vi "Dashboard Main.vi"() -> ()   [LabVIEW 2012]
uses:
  <vilib>/event_ctls.llb/eventvkey.ctl
  <vilib>/Utility/config.llb/Read Key (String).vi
  <vilib>/Utility/config.llb/Read Key (I32).vi
  <vilib>/Utility/config.llb/Write Key (String).vi
  <vilib>/Utility/config.llb/Write Key (I32).vi
  <vilib>/Utility/config.llb/NI_LVConfig.lvlib
panel:
  out "Battery Value":dbl(slide) scale=0.0..14.0 scale format="%#_2e"
  out "Battery":sgl(graph)
  in  "Camera Settings":T1={"Frate Rate"=30, "Compression"=30, "Size"=1} {"Frate Rate" scale=1.0..30.0; "Size" items=["640x480", "320x240", "160x120"]}
  out "Mode":T2(ring)=enum."Auto Disabled"
  out "Camera IP":string
  out "JS1 Z":dbl(slide) scale=-1.0..1.0 scale format="%#_2e"
  out "JS2 Z":dbl(slide) scale=-1.0..1.0 scale format="%#_2e"
  out "Joystick 1":cluster{"X":dbl, "Y":dbl}[](graph)
  out "Joystick 2":cluster{"X":dbl, "Y":dbl}[](graph)
  out "JS Buttons 1":T3
  out "JS Buttons 2":T3
  out "MotorSlide4":dbl(slide) scale=-1.0..1.0 scale format="%#_2e"
  out "MotorSlide3":dbl(slide) scale=-1.0..1.0 scale format="%#_2e"
  out "MotorSlide2":dbl(slide) scale=-1.0..1.0 scale format="%#_2e"
  in  "MotorName3":string="Front Left"
  in  "MotorName4":string="Front Right"
  in  "MotorName1":string="Rear Left"
  in  "MotorName2":string="Rear Right"
  out "MotorChart4":dbl(graph)
  out "MotorChart3":dbl(graph)
  out "MotorChart2":dbl(graph)
  out "MotorSlide1":dbl(slide) scale=-1.0..1.0 scale format="%#_2e"
  out "MotorChart1":dbl(graph)
  out "Robot IP":string
  in  "Dashboard Tab":enum32{"Operation", "Test", "Checklist"}(tab)
  in  "Fast                                                                                                             Slow 2":dbl(slide) scale=0.0..1.0
  in  "Launch Reduction\n                                                                                                             Slow":dbl(slide) scale=0.0..1.0
  in  "Field Position":enum16{"Corner", "Middle"}(ring)
  out "Left Lifter On?":bool
  out "Right Lifter On?":bool
  out "Launcher On?":bool
  in  "Slider":dbl(slide) scale=0.0..100.0 scale format="%#_3g"
  in  "On/Off":bool caption="Solenoid"
  in  "Test Name":u16(ring) items=["Select the test to run...", "Example Test", "-------------------------------", "List of tests is built in robot code.", "Replace with your own automated tests."]
  in  "Test Tree":string(tree)
  in  "Motor":cluster{"Value":dbl, "Enable":bool} {"Value" scale=-1.0..1.0 scale format="%#_3g"}
  out "Progress":T4 {"Test Progress" scale=0.0..100.0}
  in  "Rev/Fwd":cluster{"Forward":bool, "Reverse":bool}
  in  "Ring":u16(ring) items=["Auto", "Fixed indoor", "Fixed outdoor 1", "Fixed outdoor 2", "Fixed fluorescent 1", "Fixed fluorescent 2", "Hold current"]
  in  "Listbox":i32(listbox)
  in  "Viewer":T5(tab)
  out "Mbps":dbl format="%#.1g"
  in  "Enable":bool=TRUE
  in  "DB Camera Config":bool
  out "Mbps":bool
  out "fps":dbl format="%#.1g"
  out "Image Error Message":string="Timeout in Camera Communications"
  out "Camera Image":T6(plugin-control)
  out "Buttons 1":cluster{"1":bool, "2":bool, "3":bool}
  out "Kinect 1":cluster{"X":dbl, "Y":dbl, "Z":dbl} {"X" scale=1.0..-1.0; "Y" scale=1.0..-1.0; "Z" scale=1.0..-1.0}
  out "Buttons 2":cluster{"1":bool, "2":bool, "3":bool}
  out "Kinect 2":cluster{"X":dbl, "Y":dbl, "Z":dbl} {"X" scale=1.0..-1.0; "Y" scale=1.0..-1.0; "Z" scale=1.0..-1.0}
  out "Version":string
  out "Skeleton Picture":picture
  out "Players":i8
  out "Tree":string(tree)
  # "Drive & Motors"
  # "Robot IP:"
  # "Launch Reduction"
  # "Auton Launch Reduction"
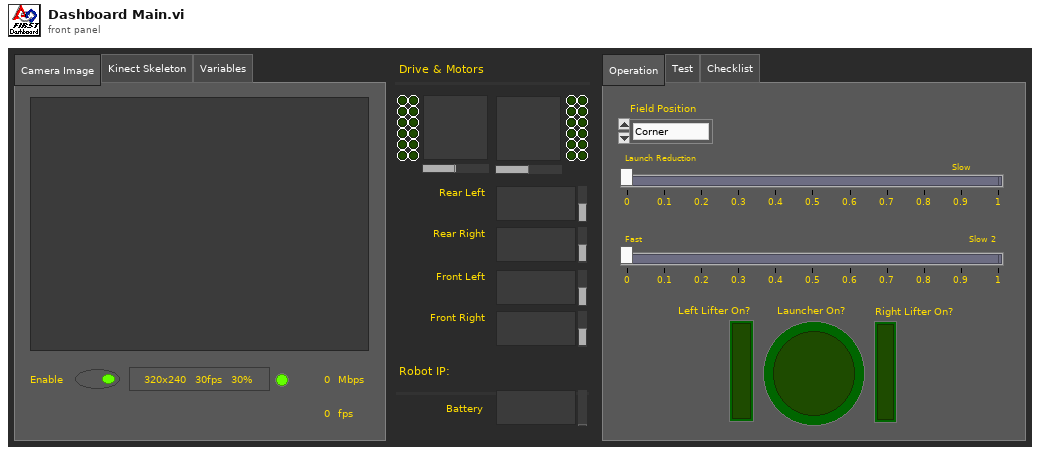
[diagram p1: front panel]
types:
  T1 = cluster{"Frate Rate":i32, "Compression":i32, "Size":u16}
  T2 = enum8{"Tele-Op Disabled", "Tele-Op Enabled", "Auto Disabled", "Auto Enabled", "Test Disabled", "Test Enabled", ""}
  T3 = cluster{bool, bool, bool, bool, bool, bool, bool, bool, bool, bool, bool, bool}
  T4 = cluster{"Test Progress":u8, "Test Progress Text":string}
  T5 = enum32{"Camera Image", "Kinect Skeleton", "Variables"}
  T6 = typedef "IMAQ Image.ctl" = refnum<image>
  T7 = typedef "Image Type" = u32
  T8 = typedef "LVBoundsTypeDef.ctl" = cluster{"Width":u32, "Height":u32}
  T9 = typedef "SkeletonTrackState.ctl" = enum32{"NotTracked", "PositionOnly", "Tracked"}
  T10 = cluster{"TrackingState":u8[], "Position":cluster{"x":sgl, "y":sgl, "z":sgl}, cluster{"x":sgl, "y":sgl, "z":sgl, sgl}[], "TrackState":T9}
  T11 = cluster{cluster{"ScaledToPercentRange":dbl, "ScaledToPercentRange":dbl, "ScaledToPercentRange":dbl}, cluster{bool, bool, bool}}[]
  T12 = cluster{cluster{"ScaledToPercentRange":dbl, "ScaledToPercentRange":dbl, "ScaledToPercentRange":dbl}, cluster{bool, bool, bool}}
  T13 = cluster{"ScaledToPercentRange":dbl, "ScaledToPercentRange":dbl, "ScaledToPercentRange":dbl}
  T14 = typedef "LVRectTypeDef.ctl" = cluster{"Left":i16, "Top":i16, "Right":i16, "Bottom":i16}
  T15 = typedef "NI_LVConfig.lvlib/Config Data RefNum.ctl" = refnum<k1>
  T16 = cluster{"Competition mode":bool, "Robot Link":bool, "Autonomous":bool, "Enabled":bool, "E-Stop":bool, "Simulated":bool, "TestMode":bool, "Docked Window":bool}
  T17 = cluster{"Boolean Array[0]":bool, "Boolean Array[1]":bool, "Boolean Array[2]":bool, "Boolean Array[3]":bool, "Boolean Array[4]":bool, "Boolean Array[5]":bool, "Boolean Array[6]":bool, "Boolean Array[7]":bool, "Boolean Array[8]":bool, "Boolean Array[9]":bool, "Boolean Array[10]":bool, "Boolean Array[11]":bool}
  T18 = typedef "eventvkey.ctl" = enum16{"ASCII", "Enter", "Return", "Shift", "Ctrl", "Alt", "Cmd", "Opt", "Caps", "NumLock", "Clear", "Break", "Up", "Down", "Left", "Right", "Insert", "Delete", "Home", "End", "PageUp", "PageDown", "Escape", "Help", "Pause", "ScrollLock", "F1", "F2", "F3", "F4", "F5", "F6", "F7", "F8", "F9", "F10", "F11", "F12", "F13", "F14", "F15", "F16", "F17", "F18", "F19", "F20", "F21", "F22", "F23", "F24", "Play", "VolumeUp", "VolumeDown", "Mute", "Two Byte Char"}
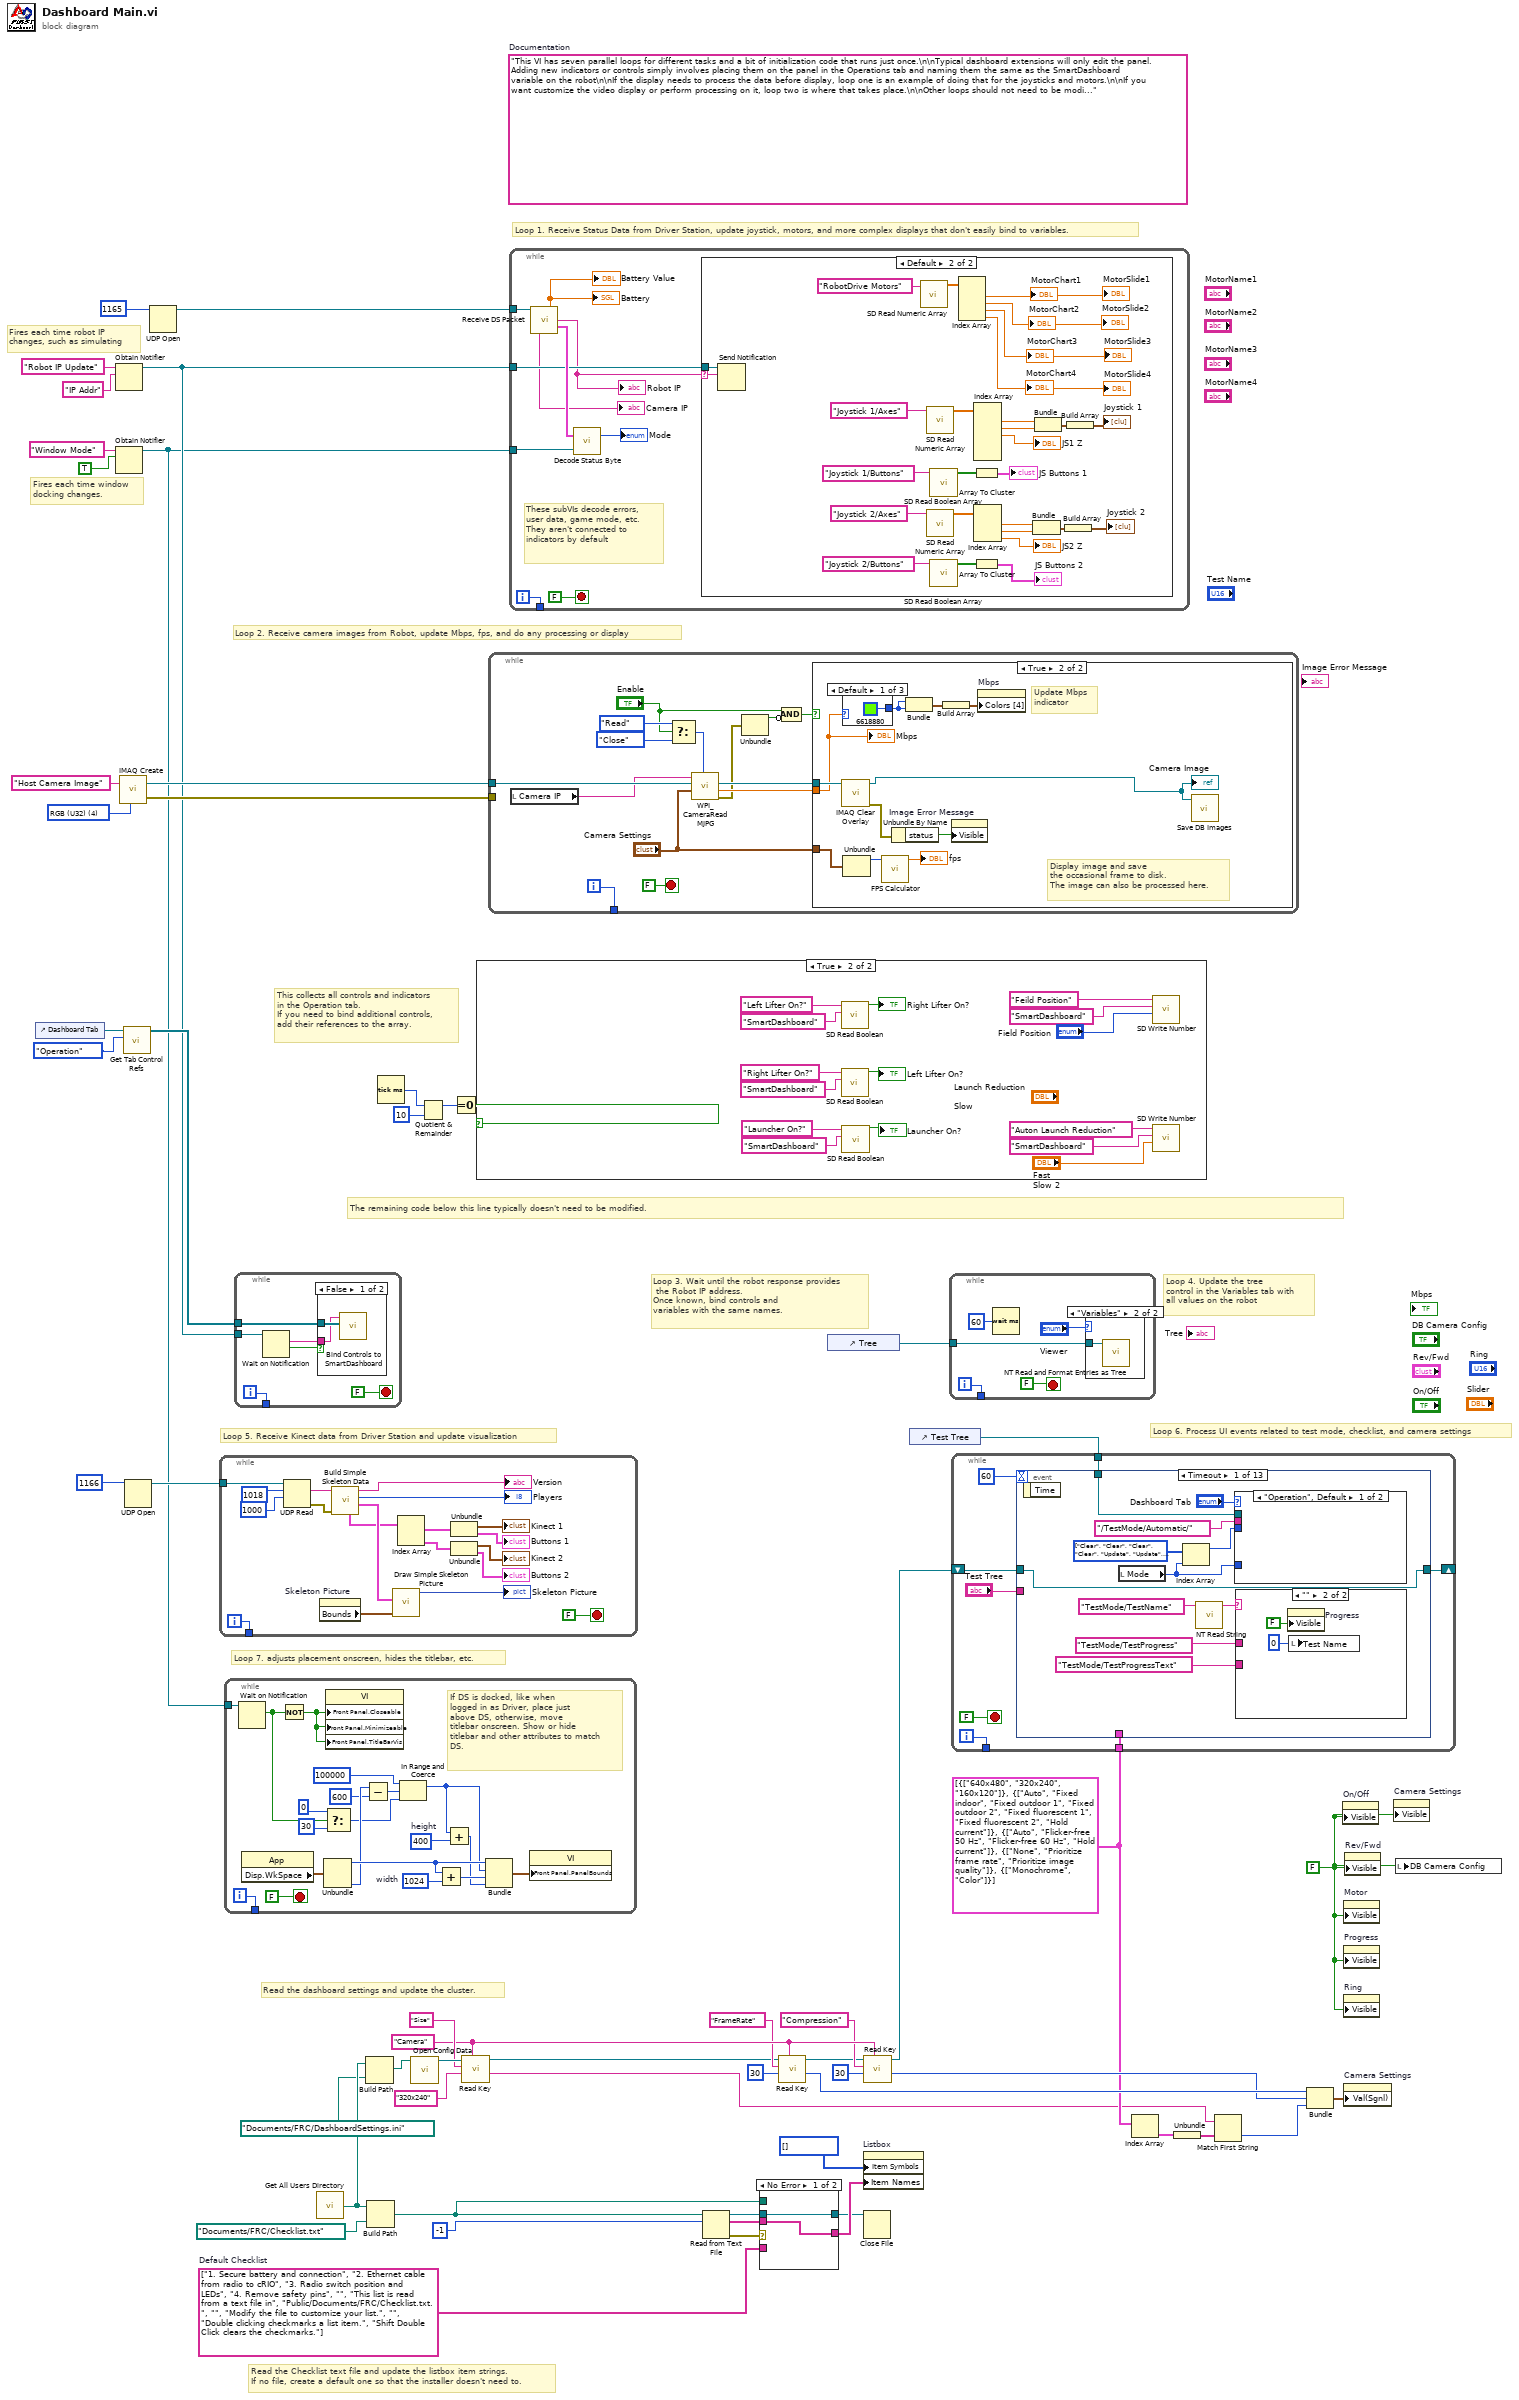
[diagram p0: block diagram]
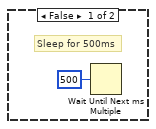
[diagram p4: hidden frame]
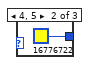
[diagram p5: hidden frame]
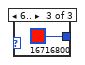
[diagram p6: hidden frame]
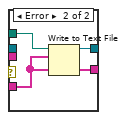
[diagram p7: hidden frame]
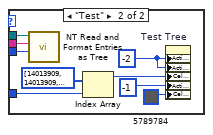
[diagram p8: hidden frame]
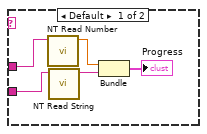
[diagram p9: hidden frame]
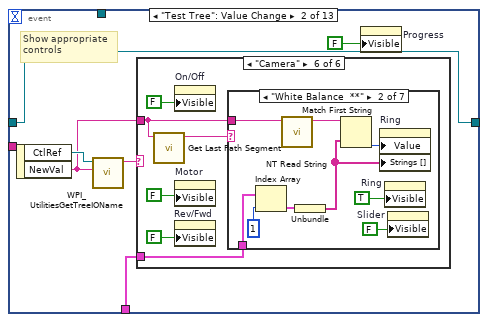
[diagram p10: hidden frame]
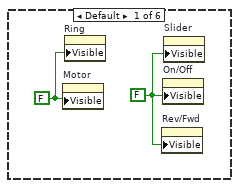
[diagram p11: hidden frame]
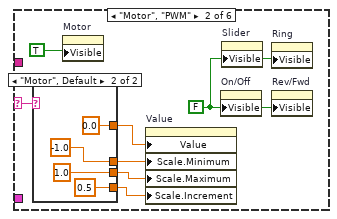
[diagram p12: hidden frame]
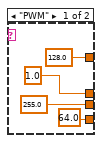
[diagram p13: hidden frame]
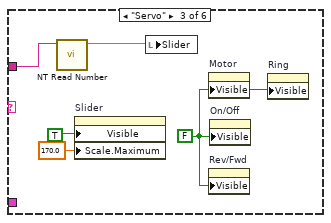
[diagram p14: hidden frame]
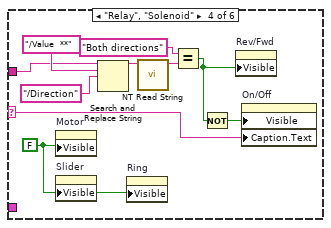
[diagram p15: hidden frame]
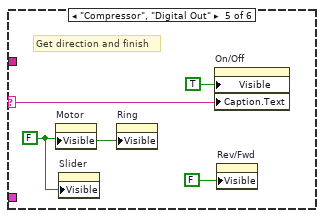
[diagram p16: hidden frame]
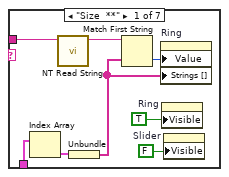
[diagram p17: hidden frame]
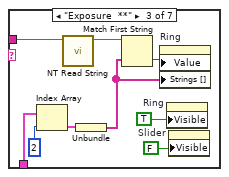
[diagram p18: hidden frame]
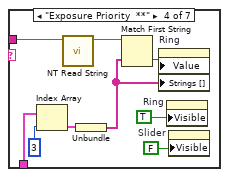
[diagram p19: hidden frame]
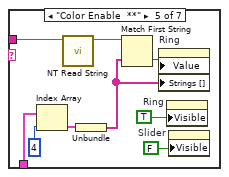
[diagram p20: hidden frame]
diagram:
  w25 = "Camera"
  w17 = cluster{string[]}[] [{["640x480", "320x240", "160x120"]}, {["Auto", "Fixed indoor", "Fixed outdoor 1", "Fixed outdoor 2", "Fixed fluorescent 1", "Fixed fluorescent 2", "Hold current"]}, {["Auto", "Flicker-free 50 Hz", "Flicker-free 60 Hz", "Hold current"]}, {["None", "Prioritize frame rate", "Prioritize image quality"]}, {["Monochrome", "Color"]}]
  w33 = string[] ["1. Secure battery and connection", "2. Ethernet cable from radio to cRIO", "3. Radio switch position and LEDs", "4. Remove safety pins", "", "This list is read from a text file in", "Public/Documents/FRC/Checklist.txt.", "", "Modify the file to customize your list.", "", "Double clicking checkmarks a list item.", "Shift Double Click clears the checkmarks."]  # Default Checklist
  w31 = FALSE ("Visible")
  (unwired) "This VI has seven parallel loops for different tasks and a bit of initialization code that runs just once.\n\nTypical dashboard extensions will only edit the panel. Adding new indicators or controls simply involves placing them on the panel in the Operations tab and naming them the same as the SmartDashboard variable on the robot\n\nIf the display needs to process the data before display, loop one is an example of doing that for the joysticks and motors.\n\nIf you want customize the video display or perform processing on it, loop two is where that takes place.\n\nOther loops should not need to be modified. They are pretty standard, and document the task they perform."  # Documentation
  w54 = T7 4 items=["Grayscale (U8)", "Grayscale (I16)", "Grayscale (SGL)", "Complex (CSG)", "RGB (U32)", "HSL (U32)", "RGB (U64)"] ("Image Type")
  # "Fires each time robot IP\nchanges, such as simulating"
  # "Fires each time window\ndocking changes."
  # "Read the Checklist text file and update the listbox item strings.\nIf no file, create a default one so that the installer doesn't need to."
  # "This collects all controls and indicators\nin the Operation tab.\nIf you need to bind additional controls,\nadd their references to the array."
  # "The remaining code below this line typically doesn't need to be modified."
  # "Loop 6. Process UI events related to test mode, checklist, and camera settings"
  # "Read the dashboard settings and update the cluster."
  # "Loop 4. Update the tree\ncontrol in the Variables tab with\nall values on the robot"
  # "Loop 3. Wait until the robot response provides\n the Robot IP address.\nOnce known, bind controls and\nvariables with the same names."
  # "Loop 5. Receive Kinect data from Driver Station and update visualization"
  # "Loop 7. adjusts placement onscreen, hides the titlebar, etc."
  # "Loop 1. Receive Status Data from Driver Station, update joystick, motors, and more complex displays that don't easily bind to variables."
  # "Loop 2. Receive camera images from Robot, update Mbps, fps, and do any processing or display"
  n1 = control-ref of="Dashboard Tab"() -> (w47:refnum<vi>)
  n2 = Obtain Notifier(name (unnamed)="Robot IP Update", notification data type="IP Addr" ("name (unnamed)")) -> (notifier out=w44:refnum<notifier>)  [unwired: 2 in, 2 out]
  n3 = Obtain Notifier(name (unnamed)="Window Mode", notification data type=TRUE) -> (notifier out=w37:refnum<notifier>)  [unwired: 2 in, 2 out]
  n4 = call "IMAQ Create"("Image Name"="Host Camera Image", "Image Type"=w54) -> ("New Image"=w52:T6, "error out"=w51:errorcluster)  [unwired: 2 in, 1 out]
  n5 = call <vilib>:"Get Tab Control Refs.vi"("Page Index"=enum32{"Operation", "Test"}."Operation" ("Dashboard Tab"), "TabControl in"=w47) -> ("ControlsOnPage"=w48:refnum<vi>[])  [unwired: 9 in]
  n6 = UDP Open(11:u16 1166 ("port")) -> (port=w49:refnum<k16>)  [unwired: 2 in, 4 out]
  n7 = UDP Open(11:u16 1165 ("port")) -> (port=w55:refnum<k16>)  [unwired: 2 in, 4 out]
  n8 = while {
    tunnel: w49 -> [w73]
    tunnel: [w58] -> _
    i -> [w58]
    stop <- FALSE stop-if-true
    n9 = UDP Read(connection ID=w73, max size (548)=1018 ("bytes to read"), timeout ms (25000)=1000) -> (data out=w67:string, error out=w57:errorcluster)  [unwired: 1 in, 3 out]
    n10 = property on="Skeleton Picture" class="Pict"() -> ("Bounds"=w69:T8)  [unwired: 2 in, 2 out]
    n11 = call "Build Simple Skeleton Data.vi"("error in (no error)"=w57, "data in"=w67) -> ("Skeleton Data"=w68:T10, "NumPlayers"=→"Players":i8, "Version String"=→"Version":string, "Simple Joystick Info"=w65:T11)  [unwired: 5 in, 1 out]
    n12 = call "Draw Simple Skeleton Picture.vi"("Bounds"=w69, "Simple Skeleton"=w68) -> ("new picture out"=→"Skeleton Picture":picture)  [unwired: 9 in]
    n13 = Index Array(array=w65) -> (element #1=w64:T12, element #2=w63:T12)  [unwired: 2 in]
    n14 = Unbundle(w64) -> (→"Kinect 1":T13, →"Buttons 1":cluster{bool, bool, bool})
    n15 = Unbundle(w63) -> (→"Kinect 2":T13, →"Buttons 2":cluster{bool, bool, bool})
  }
  n16 = while {
    tunnel: w37 -> [w94]
    tunnel: [w92] -> _
    i -> [w92]
    stop <- FALSE stop-if-true
    w84 = 1024  # width
    w87 = 400  # height
    # "If DS is docked, like when\nlogged in as Driver, place just\nabove DS, otherwise, move\ntitlebar onscreen. Show or hide\ntitlebar and other attributes to match\nDS."
    n17 = Wait on Notification(notifier=w94) -> (notification=w79:bool)  [unwired: 3 in, 3 out]
    n18 = property class="App"() -> ("Disp.WkSpace"=w90:T14)  [unwired: 2 in, 2 out]
    n19 = Not(x=w79) -> (.not. x?=w93:bool)
    n20 = Unbundle(w90) -> ("Left"=w88:i16, "Bottom"=w85:i16)  [unwired: 2 out]
    n21 = Select(t=0, s=w79, f=30) -> (s? t:f=w78:i32)
    n22 = property class="VI"("Front Panel.Closeable"=w93, "Front Panel.Minimizeable"=w93, "Front Panel.TitleBarVis"=w93) -> ()  [unwired: 2 in, 2 out]
    n23 = Subtract(x=w85, y=600) -> (x-y=w82:i32)
    n24 = In Range and Coerce(upper limit=100000, x=w82, lower limit=w78) -> (coerced(x)=w76:i32)  [unwired: 1 out]
    n25 = Add(x=w88, y=w84) -> (x+y=w89:i32)
    n26 = Add(x=w76, y=w87) -> (x+y=w86:i32)
    n27 = Bundle("Left"=w88, w76, w89, w86) -> (w91:cluster{"Left":i16, i32, i32, i32})  [unwired: 1 out]
    n28 = property class="VI"("Front Panel.PanelBounds"=w91) -> ()  [unwired: 2 in, 2 out]
  }
  n29 = while {
    tunnel: w48 -> [w101]
    tunnel: w44 -> [w98]
    tunnel: [w96] -> _
    i -> [w96]
    stop <- FALSE stop-if-true
    n30 = Wait on Notification(notifier=w98) -> (notification=w97:string, timed out?=w99:bool)  [unwired: 3 in, 2 out]
    n31 = case shown="False" w99 {
      tunnel: w101 -> [w103 _]
      tunnel: w97 -> [w102 _]
      frame False {
        n32 = call <vilib>:"Bind Controls to SmartDashboard.vi"("Bound Control Refs"=w103, "Server IP Address"=w102) -> ()  [unwired: 10 in]
      }
      frame True {
      }
    }
  }
  n33 = call "Get All Users Directory.vi"() -> ("All User Path"=w30:path)
  n34 = Build Path(base path=w30, name or relative path=path "Documents/FRC/DashboardSettings.ini") -> (appended path=w29:path)
  n35 = Build Path(base path=w30, name or relative path=path "Documents/FRC/Checklist.txt") -> (appended path=w34:path)
  n36 = Tick Count (ms)() -> (millisecond timer value=w4:u32)
  n37 = call <vilib>:"Open Config Data.vi"("configuration file path"=w29) -> ("refnum"=w28:T15)  [unwired: 8 in, 2 out]
  n38 = Quotient & Remainder(x=w4, y=u32 10) -> (x-y*floor(x/y)=w2:u32)  [unwired: 1 out]
  n39 = Equal To 0?(x=w2) -> (x = 0?=w1:bool)
  n40 = call-poly <vilib>:"Read Key.vi"("section"=w25, "default value"="320x240", "key"="Size", "refnum"=w28) -> ("value"=w15:string, "refnum out"=w10:T15)  [unwired: 2 in, 4 out]
  n41 = case shown="True" w1 {
    frame False {
    }
    frame True {
      n42 = call <vilib>:"SD Read Boolean.vi"("Table Prefix"="SmartDashboard", "Name"="Left Lifter On?") -> ("Boolean"=→"Right Lifter On?":bool)  [unwired: 7 in, 2 out]
      n43 = call <vilib>:"SD Read Boolean.vi"("Table Prefix"="SmartDashboard", "Name"="Right Lifter On?") -> ("Boolean"=→"Left Lifter On?":bool)  [unwired: 7 in, 2 out]
      n44 = call <vilib>:"SD Read Boolean.vi"("Table Prefix"="SmartDashboard", "Name"="Launcher On?") -> ("Boolean"=→"Launcher On?":bool)  [unwired: 7 in, 2 out]
      n45 = call <vilib>:"SD Write Number.vi"("Numeric"="Field Position", "Table Prefix"="SmartDashboard", "Name"="Feild Position") -> ()  [unwired: 7 in, 2 out]
      n46 = call <vilib>:"SD Write Number.vi"("Numeric"="Fast                                                                                                             Slow 2", "Table Prefix"="SmartDashboard", "Name"="Auton Launch Reduction") -> ()  [unwired: 7 in, 2 out]
    }
  }
  n47 = while {
    tunnel: w52 -> [w122]
    tunnel: w51 -> [_]
    tunnel: [w131] -> _
    i -> [w131]
    stop <- FALSE stop-if-true
    n48 = local read "Camera IP"() -> (w119:string)
    n49 = Select(t=enum16{"Read", "Reopen", "Close"}."Read" ("Operation"), s="Enable", f=enum16{"Read", "Reopen", "Close"}."Close" ("Operation")) -> (s? t:f=w121:enum16{"Read", "Reopen", "Close"})
    n50 = call <vilib>:"WPI_CameraRead MJPG.vi"("Operation"=w121, "Camera Settings"="Camera Settings", "Image"=w122, "address"=w119) -> ("error out"=w126:errorcluster, "Bandwidth (kbps)"=w128:dbl, "Image Out"=w129:T6)  [unwired: 5 in]
    n51 = Unbundle(w126) -> ("status"=w124:bool)  [unwired: 2 out]
    n52 = Compound Arithmetic op=AND("Enable", invert w124) -> (w123:bool)
    n53 = case shown="True" w123 {
      tunnel: "Camera Settings" -> [_ w136]
      tunnel: w129 -> [_ w139]
      tunnel: w128 -> [_ w138]
      frame False {
        # "Sleep for 500ms"
        n54 = Wait Until Next ms Multiple(millisecond multiple=u32 500) -> ()  [unwired: 1 out]
      }
      frame True {
        # "Display image and save\nthe occasional frame to disk.\nThe image can also be processed here."
        # "Update Mbps\nindicator"
        n55 = call "IMAQ Clear Overlay"("Image"=w139) -> ("error out"=w143:errorcluster, "Image Out"=w134:T6)  [unwired: 2 in, 7 out]
        "Camera Image" <- w134
        n56 = case shown="Default" w138 {
          tunnel: [u32 6618880 ("Color Box") u32 16776722 ("Color Box") u32 16716800 ("Color Box")] -> w140
          frame Default {
          }
          frame 4, 5 {
          }
          frame 6.. {
          }
        }
        n57 = Unbundle(w136) -> ("Frate Rate"=w135:i32)  [unwired: 2 out]
        n58 = call "FPS Calculator.vi"("Average Count"=w135) -> ("fps"=→"fps":dbl)  [unwired: 10 in]
        n59 = Unbundle By Name(w143) -> ("status"=w144:bool)
        n60 = Bundle("Color Box"=w140, "Color Box"=w140) -> (w142:cluster{"Color Box":u32, "Color Box":u32})  [unwired: 1 out]
        n61 = Build Array(w142) -> (w141:cluster{"Color Box":u32, "Color Box":u32}[])
        n62 = property on="Image Error Message" class="Str"("Visible"=w144) -> ()  [unwired: 2 in, 2 out]
        n63 = property on="Mbps" class="Bool (strict)"("Colors [4]"=w141) -> ()  [unwired: 2 in, 2 out]
        n64 = call "Save DB Images.vi"("Image"=w134) -> ()  [unwired: 2 in, 1 out]
        "Mbps" <- w138
      }
    }
  }
  n65 = while {
    tunnel: w55 -> [w155]
    tunnel: w44 -> [w150]
    tunnel: w37 -> [w153]
    tunnel: [w151] -> _
    i -> [w151]
    stop <- FALSE stop-if-true
    # "These subVIs decode errors, user data, game mode, etc.\nThey aren't connected to indicators by default"
    n66 = call "Receive DS Packet.vi"("Recv Socket"=w155) -> ("Battery"=→"Battery" →"Battery Value":sgl, "Robot IP Address"=w149:string, "Status"=w156:T16, "Camera IP Address"=→"Camera IP":string)  [unwired: 1 in, 10 out]
    "Robot IP" <- w149
    n67 = call "Decode Status Byte.vi"("Window Mode Notifier"=w153, "Status"=w156) -> ("Mode"=→"Mode":T2)  [unwired: 1 out]
    n68 = case shown="Default" w149 {
      selector: w149 -> [_ w158]
      tunnel: w150 -> [_ w159]
      frame "0.0.0.0" {
        # "Robot not responding, don't poll the variables"
      }
      frame Default {
        n69 = Send Notification(notification=w158, notifier=w159) -> ()  [unwired: 1 in, 2 out]
        n70 = call <vilib>:"SD Read Numeric Array.vi"("Name"="RobotDrive Motors") -> ("Numeric Array"=w182:dbl[])  [unwired: 8 in, 2 out]
        n71 = call <vilib>:"SD Read Numeric Array.vi"("Name"="Joystick 1/Axes") -> ("Numeric Array"=w175:dbl[])  [unwired: 8 in, 2 out]
        n72 = call <vilib>:"SD Read Numeric Array.vi"("Name"="Joystick 2/Axes") -> ("Numeric Array"=w169:dbl[])  [unwired: 8 in, 2 out]
        n73 = call <vilib>:"SD Read Boolean Array.vi"("Name"="Joystick 1/Buttons") -> ("Boolean Array"=w177:bool[])  [unwired: 8 in, 2 out]
        n74 = call <vilib>:"SD Read Boolean Array.vi"("Name"="Joystick 2/Buttons") -> ("Boolean Array"=w168:bool[])  [unwired: 8 in, 2 out]
        n75 = Index Array(array=w182) -> (element #1=→"MotorChart1" →"MotorSlide1":dbl, element #2=→"MotorSlide2" →"MotorChart2":dbl, element #3=→"MotorChart3" →"MotorSlide3":dbl, element #4=→"MotorChart4" →"MotorSlide4":dbl)  [unwired: 4 in]
        n76 = Array To Cluster(array=w177) -> (cluster=→"JS Buttons 1":T17)
        n77 = Array To Cluster(array=w168) -> (cluster=→"JS Buttons 2":T17)
        n78 = Index Array(array=w175) -> (element #1=w172:dbl, element #2=w173:dbl, element #3=→"JS1 Z":dbl)  [unwired: 6 in, 3 out]
        n79 = Index Array(array=w169) -> (element #1=w164:dbl, element #2=w163:dbl, element #3=→"JS2 Z":dbl)  [unwired: 3 in]
        n80 = Bundle("Numeric"=w164, "Numeric"=w163) -> (w165:cluster{"Numeric":dbl, "Numeric":dbl})  [unwired: 1 in]
        n81 = Bundle("Numeric"=w172, "Numeric"=w173) -> (w171:cluster{"Numeric":dbl, "Numeric":dbl})  [unwired: 1 in]
        n82 = Build Array(w165) -> (→"Joystick 2":cluster{"Numeric":dbl, "Numeric":dbl}[])
        n83 = Build Array(w171) -> (→"Joystick 1":cluster{"Numeric":dbl, "Numeric":dbl}[])
      }
    }
  }
  n84 = Read from Text File(file (use dialog)=w34, count=-1 ("timeout ms (25000)")) -> (refnum out=w12:refnum<file>, text=w35:string[], error out=w36:errorcluster)  [unwired: 2 in, 1 out]
  n85 = case shown="No Error" w36 {
    tunnel: w35 -> [w187 _]
    tunnel: [w187 w189] -> w32
    tunnel: w33 -> [_ w189]
    tunnel: w34 -> [_ w190]
    tunnel: [w186 w188] -> w11
    tunnel: w12 -> [w186 _]
    frame No Error {
    }
    frame Error {
      n86 = Write to Text File(file (use dialog)=w190, text=w189) -> (refnum out=w188:refnum<file>)  [unwired: 2 in, 2 out]
    }
  }
  n87 = call-poly <vilib>:"Read Key.vi"("section"=w25, "default value"=30, "key"="FrameRate", "refnum"=w10) -> ("value"=w20:i32, "refnum out"=w9:T15)  [unwired: 1 in, 5 out]
  n88 = control-ref of="Tree"() -> (w6:refnum<vi>)
  n89 = property on="Listbox" class="LstBox (strict)"("Item Symbols"=i32[] [], "Item Names"=w32) -> ()  [unwired: 2 in, 2 out]
  n90 = Close File(refnum=w11) -> ()  [unwired: 1 in, 2 out]
  n91 = call-poly <vilib>:"Read Key.vi"("section"=w25, "default value"=30, "key"="Compression", "refnum"=w9) -> ("value"=w19:i32, "refnum out"=w7:T15)  [unwired: 1 in, 5 out]
  n92 = control-ref of="Test Tree"() -> (w5:refnum<vi>)
  n93 = while {
    tunnel: [w192] -> _
    tunnel: w6 -> [w191]
    i -> [w192]
    stop <- FALSE stop-if-true
    n94 = Wait (ms)(milliseconds to wait=u32 60) -> ()  [unwired: 1 out]
    n95 = case shown="\"Variables\"" "Viewer" {
      tunnel: w191 -> [_ w196]
      frame Default {
      }
      frame "Variables" {
        n96 = call <vilib>:"NT Read and Format Entries as Tree.vi"("Tree Refnum"=w196) -> ()  [unwired: 9 in, 2 out]
      }
    }
  }
  n97 = while {
    tunnel: w17 -> [w201]
    shift-right: [w200] -> _
    shift-left: w7 -> [w199]
    tunnel: [w198] -> _
    tunnel: w5 -> [w197]
    i -> [w198]
    stop <- FALSE stop-if-true
    n98 = event shown="[0] Timeout" {
      selector: _ -> [_ _ _ _ _ _ _ _ _ _ _ _ _]
      dyn-events: _ -> [_ _ _ _ _ _ _ _ _ _ _ _ _]
      timeout: u32 60 ("milliseconds to wait") -> [_ _ _ _ _ _ _ _ _ _ _ _ _]
      tunnel: w197 -> [w211 _ _ _ _ _ _ _ _ _ _ _ _]
      tunnel: "Test Tree" -> [_ _ _ _ _ _ _ _ w405 w413 w415 w419 w427]
      tunnel: w201 -> [_ w233 _ _ _ _ w369 w399 _ _ _ _ _]
      tunnel: [w205 w232 _ w335 w343 w355 w368 w392 w404 w411 w414 w418 w426] -> w200
      tunnel: w199 -> [w205 w232 _ w335 w343 w355 w367 w392 w404 w411 w414 w418 w426]
      event Timeout {
        w210 = enum16{"Update", "Clear"}[] [enum."Clear", enum."Clear", enum."Clear", enum."Clear", enum."Update", enum."Update", enum."Clear"] items=["Update", "Clear"]
        n99 = event-data() -> ()  [unwired: 1 in, 1 out]
        n100 = local read "Mode"() -> (w208:T2)
        n101 = Index Array(array=w210, index=w208) -> (element=w209:enum16{"Update", "Clear"})
        n102 = call <vilib>:"NT Read String.vi"("Name"="TestMode/TestName") -> ("String"=w214:string)  [unwired: 9 in, 1 out]
        n103 = case shown="\"Operation\", Default" "Dashboard Tab" {
          tunnel: w211 -> [_ w224]
          tunnel: "/TestMode/Automatic/" ("Name Pattern") -> [_ w223]
          tunnel: w209 -> [_ w222]
          tunnel: w208 -> [_ w220]
          frame "Operation", Default {
          }
          frame "Test" {
            w219 = -2 ("Active Item:Row Number")
            n104 = call <vilib>:"NT Read and Format Entries as Tree.vi"("Operation"=w222, "Name Pattern"=w223, "Tree Refnum"=w224) -> ()  [unwired: 7 in, 2 out]
            n105 = Index Array(array=u32[] [14013909, 14013909, 14013909, 14013909, 14013909, 16777215, 14013909], index=w220) -> (element=w218:u32)
            n106 = property on="Test Tree" class="Tree (strict)"("Active Item Row Number"=w219, "ActiveColNum"=w219, "CellBG"=w218, "Active Item Row Number"=-1 ("Active Item:Row Number"), "CellBG"=u32 5789784 ("Color Box")) -> ()  [unwired: 2 in, 2 out]
          }
        }
        n107 = case shown="\"\"" w214 {
          tunnel: "TestMode/TestProgress" ("Name") -> [w226 _]
          tunnel: "TestMode/TestProgressText" ("Name") -> [w225 _]
          frame Default {
            n108 = call <vilib>:"NT Read Number.vi"("Name"=w226) -> ("Numeric"=w227:dbl)  [unwired: 9 in, 1 out]
            n109 = call <vilib>:"NT Read String.vi"("Name"=w225) -> ("String"=w228:string)  [unwired: 9 in, 1 out]
            n110 = Bundle("Numeric"=w227, "String"=w228) -> (→"Progress":cluster{"Numeric":dbl, "String":string})  [unwired: 1 in]
          }
          frame "" {
            n111 = property on="Progress" class="Clust (strict)"("Visible"=FALSE) -> ()  [unwired: 2 in, 2 out]
            n112 = local write "Test Name"(u16 0) -> ()
          }
        }
      }
      event "Test Tree": Value Change {
        # "Show appropriate\ncontrols"
        n113 = event-data() -> ("CtlRef"=w236:refnum<vi>, "NewVal"=w234:string)  [unwired: 1 in]
        n114 = call <vilib>:"WPI_UtilitiesGetTreeIOName.vi"("NewVal"=w234, "TreeControl in"=w236) -> ("I/O Name"=w237:string)  [unwired: 9 in]
        n115 = case shown="\"Camera\"" w237 {
          selector: w237 -> [_ w244 _ w262 w271 _]
          tunnel: w234 -> [_ _ w259 w261 _ w278]
          tunnel: w233 -> [_ _ _ _ _ w277]
          frame Default {
            w239 = FALSE ("Visible")
            w238 = FALSE ("Visible")
            n116 = property on="Motor" class="Clust (strict)"("Visible"=w238) -> ()  [unwired: 2 in, 2 out]
            n117 = property on="Ring" class="Ring (strict)"("Visible"=w238) -> ()  [unwired: 2 in, 2 out]
            n118 = property on="Rev/Fwd" class="Clust (strict)"("Visible"=w239) -> ()  [unwired: 2 in, 2 out]
            n119 = property on="On/Off" class="Bool (strict)"("Visible"=w239) -> ()  [unwired: 2 in, 2 out]
            n120 = property on="Slider" class="Slide (strict)"("Visible"=w239) -> ()  [unwired: 2 in, 2 out]
          }
          frame "Motor", "PWM" {
            w245 = FALSE ("Visible")
            n121 = case shown="\"Motor\", Default" w244 {
              tunnel: [1.0 ("Value") -1.0 ("Value")] -> w243
              tunnel: [255.0 ("Value") 1.0 ("Value")] -> w242
              tunnel: [128.0 ("Value") 0.0 ("Value")] -> w241
              tunnel: [64.0 ("Value") 0.5 ("Value")] -> w240
              frame "PWM" {
              }
              frame "Motor", Default {
              }
            }
            n122 = property on="Motor" class="Clust (strict)"("Visible"=TRUE) -> ()  [unwired: 2 in, 2 out]
            n123 = property on="Value" class="Slide (strict)"("Value"=w241, "Scale.Minimum"=w243, "Scale.Maximum"=w242, "Scale.Increment"=w240) -> ()  [unwired: 2 in, 2 out]
            n124 = property on="On/Off" class="Bool (strict)"("Visible"=w245) -> ()  [unwired: 2 in, 2 out]
            n125 = property on="Slider" class="Slide (strict)"("Visible"=w245) -> ()  [unwired: 2 in, 2 out]
            n126 = property on="Ring" class="Ring (strict)"("Visible"=w245) -> ()  [unwired: 2 in, 2 out]
            n127 = property on="Rev/Fwd" class="Clust (strict)"("Visible"=w245) -> ()  [unwired: 2 in, 2 out]
          }
          frame "Servo" {
            w257 = FALSE ("Visible")
            n128 = call <vilib>:"NT Read Number.vi"("Name"=w259) -> ("Numeric"=w258:dbl)  [unwired: 9 in, 1 out]
            n129 = property on="Slider" class="Slide (strict)"("Visible"=TRUE, "Scale.Maximum"=170.0 ("Scale.Range:Maximum")) -> ()  [unwired: 2 in, 2 out]
            n130 = local write "Slider"(w258) -> ()
            n131 = property on="Motor" class="Clust (strict)"("Visible"=w257) -> ()  [unwired: 2 in, 2 out]
            n132 = property on="Rev/Fwd" class="Clust (strict)"("Visible"=w257) -> ()  [unwired: 2 in, 2 out]
            n133 = property on="On/Off" class="Bool (strict)"("Visible"=w257) -> ()  [unwired: 2 in, 2 out]
            n134 = property on="Ring" class="Ring (strict)"("Visible"=w257) -> ()  [unwired: 2 in, 2 out]
          }
          frame "Relay", "Solenoid" {
            w260 = FALSE ("Visible")
            n135 = property on="Motor" class="Clust (strict)"("Visible"=w260) -> ()  [unwired: 2 in, 2 out]
            n136 = property on="Slider" class="Slide (strict)"("Visible"=w260) -> ()  [unwired: 2 in, 2 out]
            n137 = Search and Replace String(input string=w261, search string="/Value  **", replace string="/Direction") -> (result string=w267:string)  [unwired: 5 in, 3 out]
            n138 = property on="Ring" class="Ring (strict)"("Visible"=w260) -> ()  [unwired: 2 in, 2 out]
            n139 = call <vilib>:"NT Read String.vi"("Name"=w267) -> ("String"=w265:string)  [unwired: 9 in, 1 out]
            n140 = Equal?(x="Both directions", y=w265) -> (x = y?=w263:bool)
            n141 = Not(x=w263) -> (.not. x?=w264:bool)
            n142 = property on="Rev/Fwd" class="Clust (strict)"("Visible"=w263) -> ()  [unwired: 2 in, 2 out]
            n143 = property on="On/Off" class="Bool (strict)"("Visible"=w264, "Caption.Text"=w262) -> ()  [unwired: 2 in, 2 out]
          }
          frame "Compressor", "Digital Out" {
            w270 = FALSE ("Visible")
            # "Get direction and finish"
            n144 = property on="Motor" class="Clust (strict)"("Visible"=w270) -> ()  [unwired: 2 in, 2 out]
            n145 = property on="Slider" class="Slide (strict)"("Visible"=w270) -> ()  [unwired: 2 in, 2 out]
            n146 = property on="Ring" class="Ring (strict)"("Visible"=w270) -> ()  [unwired: 2 in, 2 out]
            n147 = property on="On/Off" class="Bool (strict)"("Visible"=TRUE, "Caption.Text"=w271) -> ()  [unwired: 2 in, 2 out]
            n148 = property on="Rev/Fwd" class="Clust (strict)"("Visible"=FALSE) -> ()  [unwired: 2 in, 2 out]
          }
          frame "Camera" {
            n149 = call <vilib>:"Get Last Path Segment.vi"("String in"=w278) -> ("String out"=w279:string)  [unwired: 10 in]
            n150 = property on="On/Off" class="Bool (strict)"("Visible"=FALSE) -> ()  [unwired: 2 in, 2 out]
            n151 = property on="Motor" class="Clust (strict)"("Visible"=FALSE) -> ()  [unwired: 2 in, 2 out]
            n152 = property on="Rev/Fwd" class="Clust (strict)"("Visible"=FALSE) -> ()  [unwired: 2 in, 2 out]
            n153 = case shown="\"White Balance  **\"" w279 {
              tunnel: w278 -> [w285 w294 w303 w312 w321 _ w327]
              tunnel: w277 -> [w283 w291 w300 w309 w318 _ _]
              frame "Size  **" {
                n154 = Index Array(array=w283) -> (element=w282:cluster{string[]})  [unwired: 1 in]
                n155 = call <vilib>:"NT Read String.vi"("Name"=w285) -> ("String"=w284:string)  [unwired: 9 in, 1 out]
                n156 = Unbundle(w282) -> (w280:string[])
                n157 = Match First String(2:w280, 3:w284) -> (0:w281:i32)  [unwired: 1 out]
                n158 = property on="Ring" class="Ring (strict)"("Value"=w281, "Strings []"=w280) -> ()  [unwired: 2 in, 2 out]
                n159 = property on="Ring" class="Ring (strict)"("Visible"=TRUE) -> ()  [unwired: 2 in, 2 out]
                n160 = property on="Slider" class="Slide (strict)"("Visible"=FALSE) -> ()  [unwired: 2 in, 2 out]
              }
              frame "White Balance  **" {
                n161 = Index Array(array=w291, index=1) -> (element=w292:cluster{string[]})
                n162 = call <vilib>:"NT Read String.vi"("Name"=w294) -> ("String"=w293:string)  [unwired: 9 in, 1 out]
                n163 = Unbundle(w292) -> (w289:string[])
                n164 = Match First String(2:w289, 3:w293) -> (0:w288:i32)  [unwired: 1 out]
                n165 = property on="Ring" class="Ring (strict)"("Value"=w288, "Strings []"=w289) -> ()  [unwired: 2 in, 2 out]
                n166 = property on="Ring" class="Ring (strict)"("Visible"=TRUE) -> ()  [unwired: 2 in, 2 out]
                n167 = property on="Slider" class="Slide (strict)"("Visible"=FALSE) -> ()  [unwired: 2 in, 2 out]
              }
              frame "Exposure  **" {
                n168 = Index Array(array=w300, index=2) -> (element=w301:cluster{string[]})
                n169 = call <vilib>:"NT Read String.vi"("Name"=w303) -> ("String"=w302:string)  [unwired: 9 in, 1 out]
                n170 = Unbundle(w301) -> (w297:string[])
                n171 = Match First String(2:w297, 3:w302) -> (0:w298:i32)  [unwired: 1 out]
                n172 = property on="Ring" class="Ring (strict)"("Value"=w298, "Strings []"=w297) -> ()  [unwired: 2 in, 2 out]
                n173 = property on="Ring" class="Ring (strict)"("Visible"=TRUE) -> ()  [unwired: 2 in, 2 out]
                n174 = property on="Slider" class="Slide (strict)"("Visible"=FALSE) -> ()  [unwired: 2 in, 2 out]
              }
              frame "Exposure Priority  **" {
                n175 = Index Array(array=w309, index=3) -> (element=w310:cluster{string[]})
                n176 = call <vilib>:"NT Read String.vi"("Name"=w312) -> ("String"=w311:string)  [unwired: 9 in, 1 out]
                n177 = Unbundle(w310) -> (w306:string[])
                n178 = Match First String(2:w306, 3:w311) -> (0:w307:i32)  [unwired: 1 out]
                n179 = property on="Ring" class="Ring (strict)"("Value"=w307, "Strings []"=w306) -> ()  [unwired: 2 in, 2 out]
                n180 = property on="Ring" class="Ring (strict)"("Visible"=TRUE) -> ()  [unwired: 2 in, 2 out]
                n181 = property on="Slider" class="Slide (strict)"("Visible"=FALSE) -> ()  [unwired: 2 in, 2 out]
              }
              frame "Color Enable  **" {
                n182 = Index Array(array=w318, index=4) -> (element=w319:cluster{string[]})
                n183 = call <vilib>:"NT Read String.vi"("Name"=w321) -> ("String"=w320:string)  [unwired: 9 in, 1 out]
                n184 = Unbundle(w319) -> (w315:string[])
                n185 = Match First String(2:w315, 3:w320) -> (0:w316:i32)  [unwired: 1 out]
                n186 = property on="Ring" class="Ring (strict)"("Value"=w316, "Strings []"=w315) -> ()  [unwired: 2 in, 2 out]
                n187 = property on="Ring" class="Ring (strict)"("Visible"=TRUE) -> ()  [unwired: 2 in, 2 out]
                n188 = property on="Slider" class="Slide (strict)"("Visible"=FALSE) -> ()  [unwired: 2 in, 2 out]
              }
              frame Default {
                n189 = property on="Ring" class="Ring (strict)"("Visible"=FALSE) -> ()  [unwired: 2 in, 2 out]
                n190 = property on="Slider" class="Slide (strict)"("Visible"=FALSE) -> ()  [unwired: 2 in, 2 out]
              }
              frame "Brightness  **", "Color Level  **", "Compression  **", "FPS  **", "Sharpness  **" {
                n191 = call <vilib>:"NT Read Number.vi"("Name"=w327) -> ("Numeric"=w326:dbl)  [unwired: 9 in, 1 out]
                n192 = local write "Slider"(w326) -> ()
                n193 = property on="Slider" class="Slide (strict)"("Visible"=TRUE, "Scale.Maximum"=100.0 ("Scale.Range:Maximum")) -> ()  [unwired: 2 in, 2 out]
                n194 = property on="Ring" class="Ring (strict)"("Visible"=FALSE) -> ()  [unwired: 2 in, 2 out]
              }
            }
          }
        }
        n195 = property on="Progress" class="Clust (strict)"("Visible"=FALSE) -> ()  [unwired: 2 in, 2 out]
      }
      event "Test Name": Mouse Enter {
        # "Populate the ring with the list of tests"
        n196 = event-data() -> ()  [unwired: 1 in, 1 out]
        n197 = call <vilib>:"NT Read String Array.vi"("Name"="TestMode/TestList") -> ("String Array"=w334:string[])  [unwired: 9 in, 1 out]
        n198 = Build Array (concatenate)("Select the test to run...", w334) -> (w333:string[])
        n199 = property on="Test Name" class="Ring (strict)"("Strings []"=w333) -> ()  [unwired: 2 in, 2 out]
      }
      event "Test Name": Value Change {
        w336 = FALSE ("Visible")
        # "Tell the robot the test name to run"
        n200 = event-data() -> ("NewVal"=w340:u16)  [unwired: 1 in]
        n201 = property on="Test Name" class="Ring (strict)"() -> ("Strings []"=w341:string[])  [unwired: 2 in, 2 out]
        n202 = local write "Progress"(T4 {"Test Progress"=0, "Test Progress Text"=""} ("Progress")) -> ()
        n203 = Index Array(array=w341, index=w340) -> (element=w339:string)
        n204 = call <vilib>:"NT Write String.vi"("String"=w339, "Name"="TestMode/TestName") -> ()  [unwired: 9 in, 1 out]
        n205 = property on="Progress" class="Clust (strict)"("Visible"=TRUE) -> ()  [unwired: 2 in, 2 out]
        n206 = property on="Motor" class="Clust (strict)"("Visible"=w336) -> ()  [unwired: 2 in, 2 out]
        n207 = property on="Slider" class="Slide (strict)"("Visible"=w336) -> ()  [unwired: 2 in, 2 out]
        n208 = property on="On/Off" class="Bool (strict)"("Visible"=w336) -> ()  [unwired: 2 in, 2 out]
        n209 = property on="Rev/Fwd" class="Clust (strict)"("Visible"=w336) -> ()  [unwired: 2 in, 2 out]
        n210 = property on="Ring" class="Ring (strict)"("Visible"=w336) -> ()  [unwired: 2 in, 2 out]
      }
      event "Listbox": Double Click {
        n211 = event-data() -> ("PlatMods.Shift"=w344:bool, "Row"=w346:i32)  [unwired: 1 in]
        n212 = case shown="False" w344 {
          tunnel: w346 -> [w350 _]
          tunnel: 1 -> [w349 _]
          frame False {
            n213 = property on="Listbox" class="LstBox (strict)"() -> ("Item Symbols"=w348:i32[])  [unwired: 2 in, 2 out]
            n214 = Replace Array Subset(array=w348, new element=w349, index=w350) -> (w347:i32[])
            n215 = property on="Listbox" class="LstBox (strict)"("Item Symbols"=w347) -> ()  [unwired: 2 in, 2 out]
          }
          frame True {
            w351 = 0 ("Top Row")
            n216 = property on="Listbox" class="LstBox (strict)"() -> ("Number of Rows"=w353:u32)  [unwired: 2 in, 2 out]
            n217 = Initialize Array(0, w353) -> (w352:i32[])
            n218 = property on="Listbox" class="LstBox (strict)"("Top Row"=w351, "Value"=w351, "Item Symbols"=w352) -> ()  [unwired: 2 in, 2 out]
          }
        }
      }
      event "Listbox": Key Down {
        n219 = event-data() -> ("VKey"=w357:T18)  [unwired: 1 in]
        n220 = case shown="\"Left\", \"Right\"" w357 {
          selector: w357 -> [w362 _]
          tunnel: eventvkey."Left" ("VKey") -> [w360 _]
          frame "Left", "Right" {
            n221 = Equal?(x=w360, y=w362) -> (x = y?=w361:bool)
            n222 = Select(t=0, s=w361, f=1) -> (s? t:f=w363:i32)
            n223 = property on="Listbox" class="LstBox (strict)"() -> ("Item Symbols"=w366:i32[])  [unwired: 2 in, 2 out]
            n224 = Replace Array Subset(array=w366, new element=w363, index="Listbox") -> (w365:i32[])
            n225 = property on="Listbox" class="LstBox (strict)"("Item Symbols"=w365) -> ()  [unwired: 2 in, 2 out]
          }
          frame Default {
          }
        }
      }
      event "DB Camera Config": Value Change {
        n226 = event-data() -> ("NewVal"=w370:bool)  [unwired: 1 in]
        n227 = case shown="False" w370 {
          tunnel: w369 -> [w379 _]
          tunnel: [w372 w390] -> w368
          tunnel: w367 -> [w371 w390]
          frame False {
            w386 = "Camera"
            w389 = FALSE ("Visible")
            n228 = local read "Camera Settings"() -> (w378:T1)
            n229 = Index Array(array=w379) -> (element=w382:cluster{string[]})  [unwired: 1 in]
            n230 = Unbundle(w378) -> ("Frate Rate"=w377:i32, "Compression"=w376:i32, "Size"=w380:u16)
            n231 = Unbundle(w382) -> (w381:string[])
            n232 = Index Array(array=w381, index=w380) -> (element=w375:string)
            n233 = call-poly <vilib>:"Write Key.vi"("section"=w386, "value"=w375, "key"="Size", "refnum"=w371) -> ("refnum out"=w388:T15)  [unwired: 2 in, 5 out]
            n234 = call-poly <vilib>:"Write Key.vi"("section"=w386, "value"=w377, "key"="FrameRate", "refnum"=w388) -> ("refnum out"=w387:T15)  [unwired: 1 in, 6 out]
            n235 = property on="Camera Settings" class="Clust (strict)"("Visible"=w389) -> ()  [unwired: 2 in, 2 out]
            n236 = local write "DB Camera Config"(w389) -> ()
            n237 = call-poly <vilib>:"Write Key.vi"("section"=w386, "value"=w376, "key"="Compression", "refnum"=w387) -> ("refnum out"=w373:T15)  [unwired: 1 in, 6 out]
            n238 = call <vilib>:"Close Config Data.vi"("refnum"=w373) -> ("file path"=w374:path)  [unwired: 2 in, 8 out]
            n239 = call <vilib>:"Open Config Data.vi"("configuration file path"=w374) -> ("refnum"=w372:T15)  [unwired: 8 in, 2 out]
          }
          frame True {
            n240 = property on="Camera Settings" class="Clust (strict)"("Visible"=TRUE) -> ()  [unwired: 2 in, 2 out]
          }
        }
      }
      event "Camera Settings": Value Change {
        n241 = event-data() -> ("NewVal"=w403:T1)  [unwired: 1 in]
        n242 = Index Array(array=w399) -> (element=w398:cluster{string[]})  [unwired: 1 in]
        n243 = Unbundle(w403) -> ("Frate Rate"=w394:i32, "Compression"=w393:i32, "Size"=w396:u16)
        n244 = Unbundle(w398) -> (w397:string[])
        n245 = Index Array(array=w397, index=w396) -> (element=w395:string)
        n246 = Format Into String(format string="%s   %dfps   %d%%", w395, w394, w393) -> (resulting string=w400:string)  [unwired: 2 in, 1 out]
        n247 = Build Array(w400) -> (w401:string[])
        n248 = property on="DB Camera Config" class="Bool (strict)"("Strings [4]"=w401) -> ()  [unwired: 2 in, 2 out]
      }
      event "Motor.Enable": Value Change {
        n249 = event-data() -> ("NewVal"=w409:bool)  [unwired: 1 in]
        n250 = Unbundle("Motor") -> ("Value"=w408:dbl)  [unwired: 1 out]
        n251 = Select(t=w408, s=w409, f=0.0) -> (s? t:f=w406:dbl)
        n252 = call <vilib>:"NT Write Number.vi"("Numeric"=w406, "Name"=w405) -> ()  [unwired: 9 in, 1 out]
      }
      event "Slider": Value Change {
        n253 = event-data() -> ("NewVal"=w412:dbl)  [unwired: 1 in]
        n254 = call <vilib>:"NT Write Number.vi"("Numeric"=w412, "Name"=w413) -> ()  [unwired: 9 in, 1 out]
      }
      event "On/Off": Value Change {
        n255 = event-data() -> ("NewVal"=w417:bool)  [unwired: 1 in]
        n256 = Boolean To (0,1)(Boolean=w417) -> (0, 1=w416:i16)
        n257 = call <vilib>:"NT Write Number.vi"("Numeric"=w416, "Name"=w415) -> ()  [unwired: 9 in, 1 out]
      }
      event "Rev/Fwd": Value Change {
        n258 = event-data() -> ("NewVal.Forward"=w425:bool, "NewVal.Reverse"=w424:bool)  [unwired: 1 in]
        n259 = Boolean To (0,1)(Boolean=w425) -> (0, 1=w421:i16)
        n260 = Boolean To (0,1)(Boolean=w424) -> (0, 1=w423:i16)
        n261 = Negate(x=w423) -> (-x=w422:i16)
        n262 = Add(x=w421, y=w422) -> (x+y=w420:i16)
        n263 = call <vilib>:"NT Write Number.vi"("Numeric"=w420, "Name"=w419) -> ()  [unwired: 9 in, 1 out]
      }
      event "Ring": Value Change {
        n264 = event-data() -> ("NewVal"=w429:u16)  [unwired: 1 in]
        n265 = property on="Ring" class="Ring (strict)"() -> ("Strings []"=w430:string[])  [unwired: 2 in, 2 out]
        n266 = Index Array(array=w430, index=w429) -> (element=w428:string)
        n267 = call <vilib>:"NT Write String.vi"("String"=w428, "Name"=w427) -> ()  [unwired: 9 in, 1 out]
      }
    }
  }
  n268 = Index Array(array=w17) -> (element=w18:cluster{string[]})  [unwired: 1 in]
  n269 = Unbundle(w18) -> (w16:string[])
  n270 = Match First String(2:w16, 3:w15) -> (0:w14:i32)  [unwired: 1 out]
  n271 = Bundle("value"=w20, "value"=w19, "index"=w14) -> (w8:cluster{"value":i32, "value":i32, "index":i32})  [unwired: 1 out]
  n272 = property on="On/Off" class="Bool (strict)"("Visible"=w31) -> ()  [unwired: 2 in, 2 out]
  n273 = property on="Motor" class="Clust (strict)"("Visible"=w31) -> ()  [unwired: 2 in, 2 out]
  n274 = property on="Progress" class="Clust (strict)"("Visible"=w31) -> ()  [unwired: 2 in, 2 out]
  n275 = property on="Ring" class="Ring (strict)"("Visible"=w31) -> ()  [unwired: 2 in, 2 out]
  n276 = property on="Camera Settings" class="Clust (strict)"("Val(Sgnl)"=w8) -> ()  [unwired: 2 in, 2 out]
  n277 = property on="Rev/Fwd" class="Clust (strict)"("Visible"=w31) -> ()  [unwired: 2 in, 2 out]
  n278 = property on="Camera Settings" class="Clust (strict)"("Visible"=w31) -> ()  [unwired: 2 in, 2 out]
  n279 = local write "DB Camera Config"(w31) -> ()
